vi "Open-Loop Part 1.vi"() -> ()   [LabVIEW 2017]
uses:
  Pitch Array 1.ctl
  <vilib>/Analysis/coordinate.llb/Angle Units.ctl
  <vilib>/Analysis/coordinate.llb/Angle Range (Degree).ctl
  <vilib>/Analysis/coordinate.llb/Wrap Angle (scalar).vi
  <vilib>/Analysis/NI_AAL_Angle.lvlib
panel:
  out "Fan 2 Indicator":dbl(slide) scale=0.0..10.0
  out "Fan 1 Indicator":dbl(slide) scale=0.0..10.0
  in  "Bias Input":dbl(slide) scale=-25.0..25.0
  in  "Fan Power Input":dbl(slide) scale=0.0..100.0 scale format="%.2f"
  out "Pitch Angle":dbl(slide)=2.4756271011719946 scale=-80.0..80.0 scale format="%.2f"
  out "Absolute Travel Angle":dbl=11.34 format="%0.2f"
  out "Elevation Angle":dbl(slide)=26.3067514669674 scale=-50.0..50.0 scale format="%.2f"
  out "Travel Angle":dbl(knob)=11.34 scale=0.0..360.0
  in  "stop":bool
  in  "Cluster":T1={"Array"=[[80.0, 0.02, 1.0, 1.0, 1.0, 1.0, 1.0, 1.0, 1.0], [70.0, 0.11, 0.0, 0.0, 0.0, 0.0, 0.0, 0.0, 0.0], [60.0, 0.3, 0.0, 0.0, 0.0, 0.0, 0.0, 0.0, 0.0], [50.0, 0.51, 0.0, 0.0, 0.0, 0.0, 0.0, 0.0, 0.0], [40.0, 0.83, 0.0, 0.0, 0.0, 0.0, 0.0, 0.0, 0.0], [30.0, 1.13, 0.0, 0.0, 0.0, 0.0, 0.0, 0.0, 0.0], [20.0, 1.51, 0.0, 0.0, 0.0, 0.0, 0.0, 0.0, 0.0], [10.0, 2.02, 0.0, 0.0, 0.0, 0.0, 0.0, 0.0, 0.0], [0.0, 2.37, 0.0, 0.0, 0.0, 0.0, 0.0, 0.0, 0.0], [-10.0, 2.75, 0.0, 0.0, 0.0, 0.0, 0.0, 0.0, 0.0], [-20.0, 3.15, 0.0, 0.0, 0.0, 0.0, 0.0, 0.0, 0.0], [-30.0, 3.49, 0.0, 0.0, 0.0, 0.0, 0.0, 0.0, 0.0], [-40.0, 3.86, 0.0, 0.0, 0.0, 0.0, 0.0, 0.0, 0.0], [-50.0, 4.33, 0.0, 0.0, 0.0, 0.0, 0.0, 0.0, 0.0], [-60.0, 4.69, 0.0, 0.0, 0.0, 0.0, 0.0, 0.0, 0.0], [-70.0, 4.88, 0.0, 0.0, 0.0, 0.0, 0.0, 0.0, 0.0], [-80.0, 4.88, 0.0, 0.0, 0.0, 0.0, 0.0, 0.0, 0.0]], "Operation"=TRUE}
  # "Calibration\nMode"
  # "Operating\nMode"
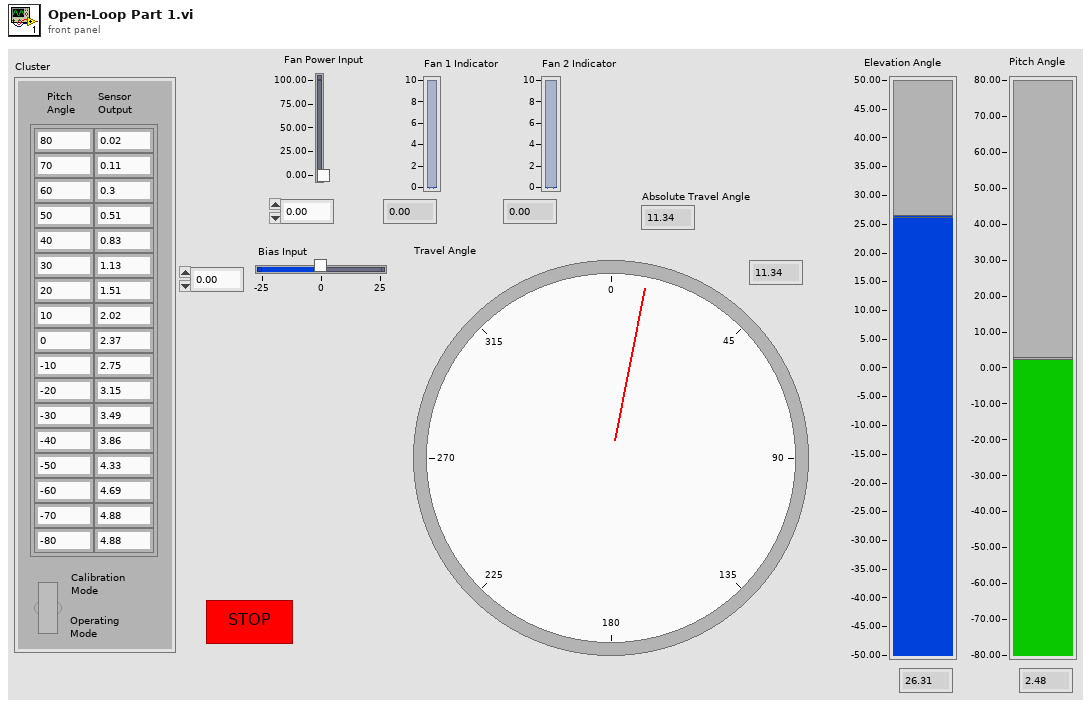
[diagram p1: front panel]
types:
  T1 = typedef "Pitch Array 1.ctl" = cluster{"Array":dbl[][], "Operation":bool}
  T2 = cluster{"AI Task":refnum<k21>, "Ctr0 Task":refnum<k21>, "Ao Task":refnum<k21>, "DO Task":refnum<k21>}
  T3 = typedef "NI_AAL_Angle.lvlib/Angle Range (Degree).ctl" = u16
  T4 = typedef "NI_AAL_Angle.lvlib/Angle Units.ctl" = i32
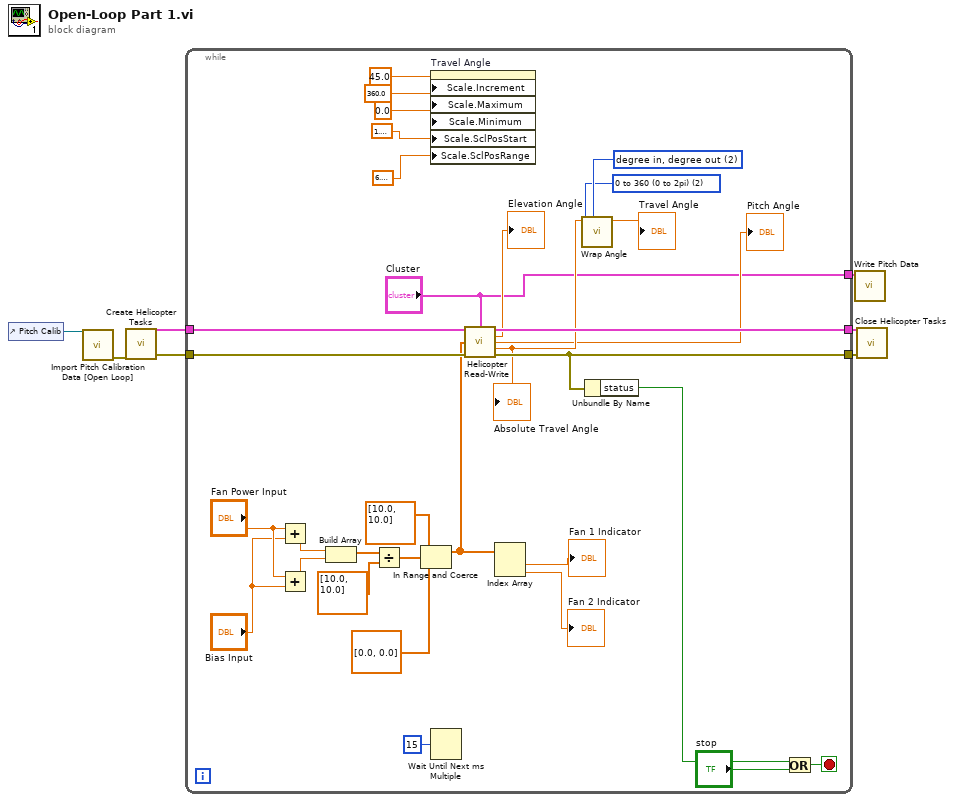
[diagram p0: block diagram]
diagram:
  n1 = control-ref of="Pitch Calib"() -> (w7:refnum<vi>)
  n2 = call "Import Pitch Calibration Data [Open Loop].vi"("Pitch Data Ref"=w7) -> ("Error Out"=w1:errorcluster)  [unwired: 10 in]
  n3 = call "Create Helicopter Tasks.vi"("Error In"=w1) -> ("Error Out"=w2:errorcluster, "Hellicopter Tasks Output"=w3:T2)  [unwired: 5 in]
  n4 = while {
    tunnel: [w37] -> w6
    tunnel: [w39] -> w5
    tunnel: ["Cluster"] -> w4
    tunnel: w3 -> [w33]
    tunnel: w2 -> [w32]
    stop <- w34 stop-if-true
    w24 = T3 2 items=["none", "-180 to 180 (-pi to pi)", "0 to 360 (0 to 2pi)"] ("angle range")
    w25 = T4 2 items=["radian in, radian out", "radian in, degree out", "degree in, degree out", "degree in, radian out"] ("angle units")
    n5 = Add(x="Fan Power Input", y="Bias Input") -> (x+y=w17:dbl)
    n6 = Add(x="Fan Power Input", y="Bias Input") -> (x+y=w16:dbl)
    n7 = Build Array(w17, w16) -> (w15:dbl[])
    n8 = Divide(x=w15, y=dbl[] [10.0, 10.0]) -> (x/y=w14:dbl[])
    n9 = In Range and Coerce(upper limit=dbl[] [10.0, 10.0], x=w14, lower limit=dbl[] [0.0, 0.0]) -> (coerced(x)=w11:dbl[])  [unwired: 1 out]
    n10 = property on="Travel Angle" class="Knob (strict)"("Scale.Increment"=45.0 ("Scale.Range:Increment"), "Scale.Maximum"=360.0 ("Scale.Range:Maximum"), "Scale.Minimum"=0.0 ("Scale.Range:Minimum"), "Scale.SclPosStart"=1.5707963267948966, "Scale.SclPosRange"=6.283185307179586) -> ()  [unwired: 2 in, 2 out]
    n11 = Wait Until Next ms Multiple(millisecond multiple=u32 15) -> ()  [unwired: 1 out]
    n12 = call "Helicopter Read-Write.vi"("Hellicopter Tasks Input"=w33, "Pitch Calib"="Cluster", "Fan Input"=w11, "Error In"=w32) -> ("Hellicopter Tasks Output"=w39:T2, "Elevation"=→"Elevation Angle":dbl, "Pitch"=→"Pitch Angle":dbl, "Travel"=w22:dbl, "Error Out"=w37:errorcluster)  [unwired: 7 in]
    "Absolute Travel Angle" <- w22
    n13 = Index Array(array=w11) -> (element #1=→"Fan 1 Indicator":dbl, element #2=→"Fan 2 Indicator":dbl)  [unwired: 2 in]
    n14 = call-poly <vilib>:"Wrap Angle.vi"("angle units"=w25, "angle range"=w24, "angle in"=w22) -> ("angle out"=→"Travel Angle":dbl)  [unwired: 7 in, 1 out]
    n15 = Unbundle By Name(w37) -> ("status"=w36:bool)
    n16 = Or(x=w36, y="stop") -> (x .or. y?=w34:bool)
  }
  n17 = call "Write Pitch Data.vi"("Pitch Calib"=w4) -> ()  [unwired: 11 in]
  n18 = call "Close Helicopter Tasks.vi"("Error In"=w6, "Hellicopter Tasks Input 2"=w5) -> ()  [unwired: 9 in, 1 out]
